vi "mirrors_and_piezo_manual_scan.vi"(1 "Stop Button":bool) -> ()   [LabVIEW 2013]
uses:
  <vilib>/Utility/error.llb/DialogType.ctl
  Piezo_micrometres_slider_control.ctl
  <vilib>/DAQmx/create/channels.llb/DAQmx Create Channel (AO-Voltage-Basic).vi
  <vilib>/DAQmx/create/channels.llb/DAQmx Create Channel (DO-Digital Output).vi
  <vilib>/DAQmx/write.llb/DAQmx Write (Analog DBL 1Chan 1Samp).vi
  <vilib>/DAQmx/write.llb/DAQmx Write (Digital Bool 1Line 1Point).vi
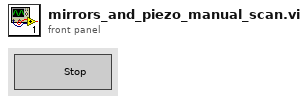
[diagram p1: front panel]
types:
  T1 = typedef "DialogType.ctl" = u16
  T2 = typedef "Piezo_micrometres_slider_control.ctl" = dbl
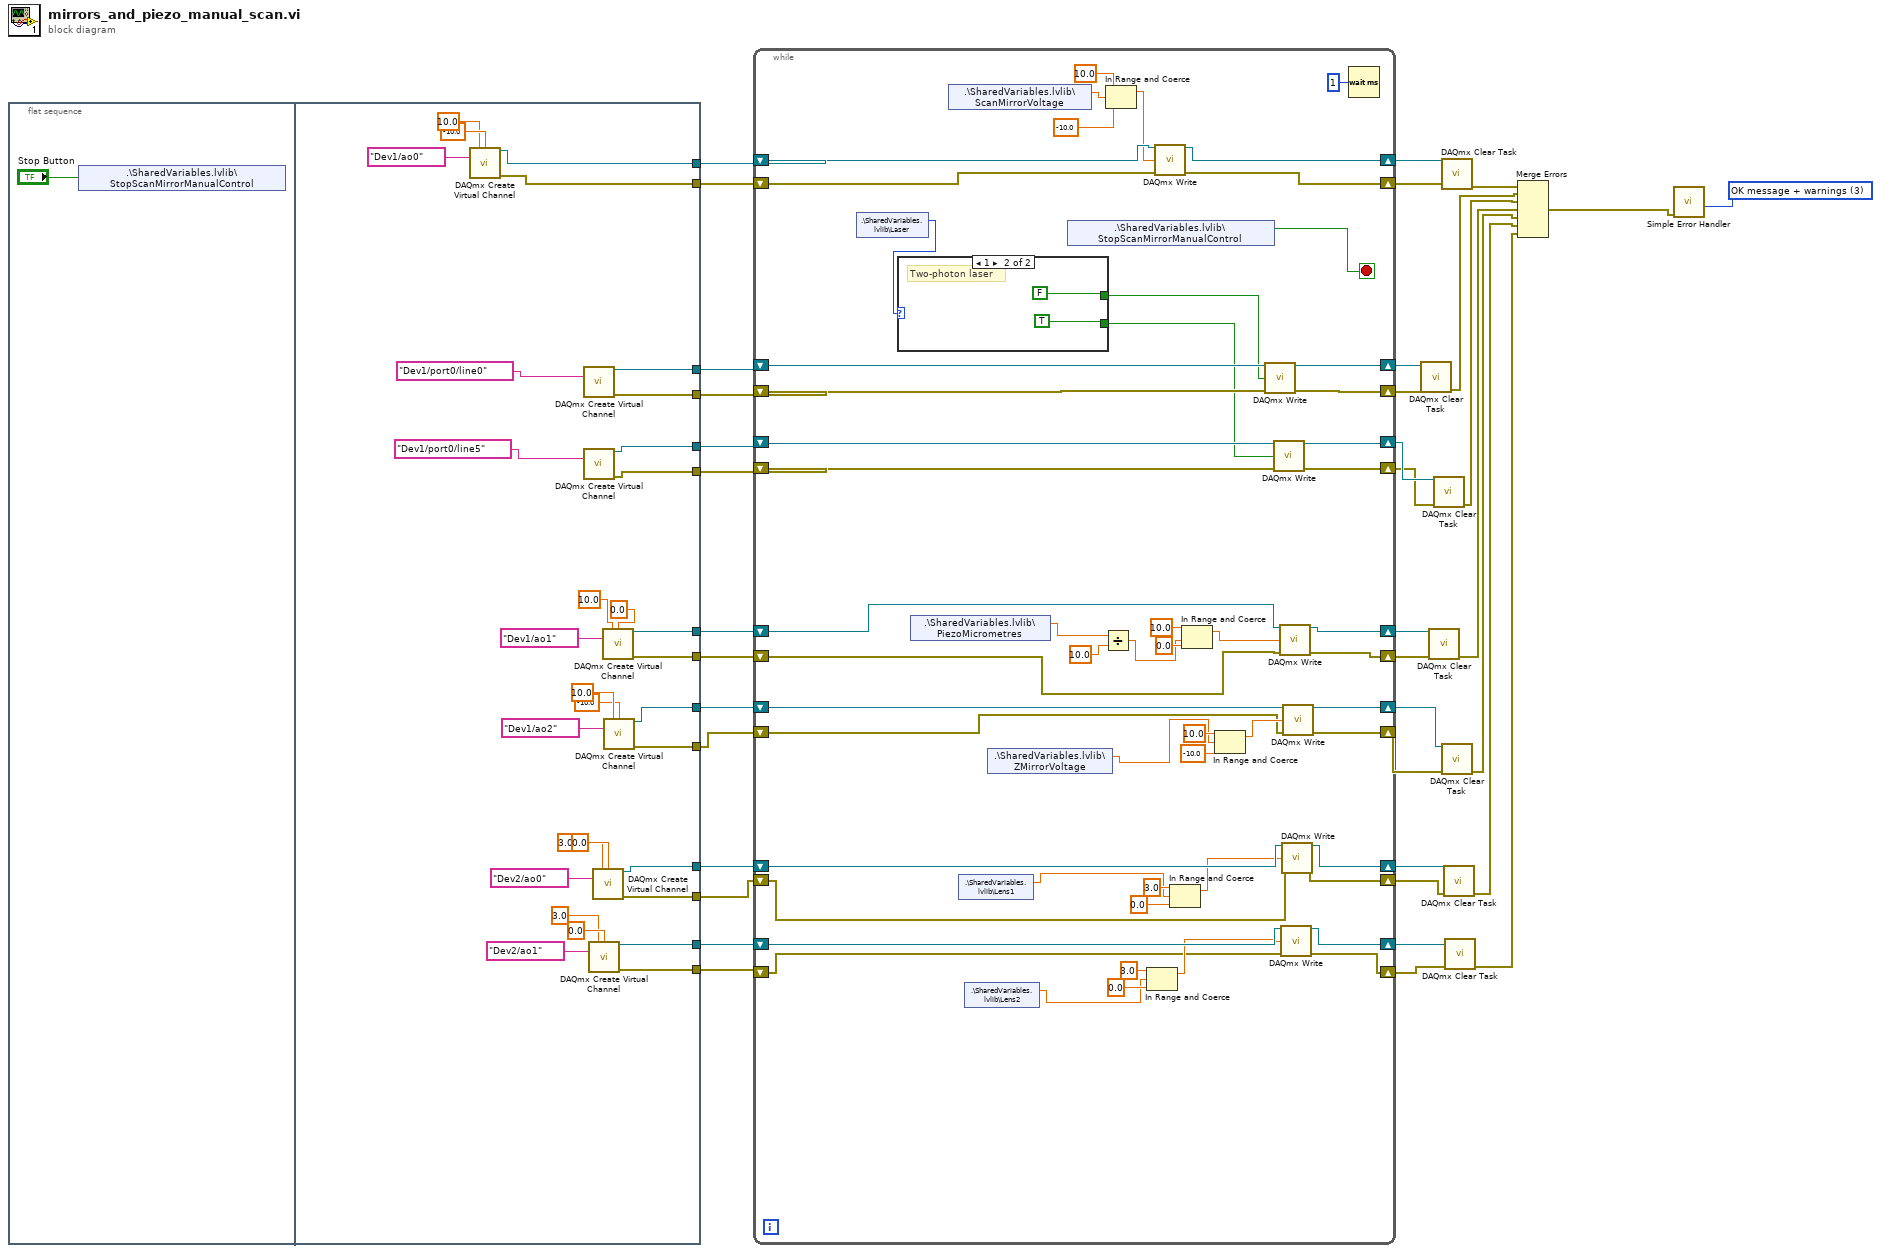
[diagram p0: block diagram]
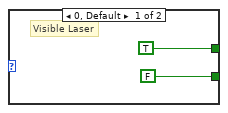
[diagram p2: hidden frame]
diagram:
  w21 = T1 3 items=["no dialog", "OK message", "continue or stop message", "OK message + warnings", "continue/stop + warnings"] ("type of dialog (OK msg:1)")
  n1 = flat-sequence {
    tunnel: [w66] -> w37
    tunnel: [w65] -> w36
    tunnel: [w64] -> w33
    tunnel: [w63] -> w32
    tunnel: [w62] -> w31
    tunnel: [w61] -> w30
    tunnel: [w52] -> w25
    tunnel: [w51] -> w24
    tunnel: [w50] -> w23
    tunnel: [w49] -> w22
    tunnel: [w48] -> w10
    tunnel: [w47] -> w5
    tunnel: [w46] -> w9
    tunnel: [w45] -> w4
    frame #0 {
      n2 = shared-variable ".\\SharedVariables.lvlib\\StopScanMirrorManualControl"("Stop Button") -> ()  [unwired: 1 in, 1 out]
    }
    frame #1 {
      n3 = call-poly <vilib>:"DAQmx Create Virtual Channel.vi"("maximum value"=10.0, "minimum value"=-10.0, "physical channels"=tag "Dev1/ao0") -> ("task out"=w66:refnum<k21>, "error out"=w65:errorcluster)  [unwired: 11 in]
      n4 = call-poly <vilib>:"DAQmx Create Virtual Channel.vi"("lines"=tag "Dev1/port0/line0" ("Physical Channel")) -> ("task out"=w64:refnum<k21>, "error out"=w63:errorcluster)  [unwired: 13 in]
      n5 = call-poly <vilib>:"DAQmx Create Virtual Channel.vi"("lines"=tag "Dev1/port0/line5") -> ("task out"=w62:refnum<k21>, "error out"=w61:errorcluster)  [unwired: 13 in]
      n6 = call-poly <vilib>:"DAQmx Create Virtual Channel.vi"("maximum value"=3.0, "minimum value"=0.0, "physical channels"=tag "Dev2/ao1") -> ("task out"=w46:refnum<k21>, "error out"=w45:errorcluster)  [unwired: 11 in]
      n7 = call-poly <vilib>:"DAQmx Create Virtual Channel.vi"("maximum value"=3.0, "minimum value"=0.0, "physical channels"=tag "Dev2/ao0") -> ("task out"=w48:refnum<k21>, "error out"=w47:errorcluster)  [unwired: 11 in]
      n8 = call-poly <vilib>:"DAQmx Create Virtual Channel.vi"("maximum value"=10.0, "minimum value"=0.0, "physical channels"=tag "Dev1/ao1") -> ("task out"=w52:refnum<k21>, "error out"=w51:errorcluster)  [unwired: 11 in]
      n9 = call-poly <vilib>:"DAQmx Create Virtual Channel.vi"("maximum value"=10.0, "minimum value"=-10.0, "physical channels"=tag "Dev1/ao2") -> ("task out"=w50:refnum<k21>, "error out"=w49:errorcluster)  [unwired: 11 in]
    }
  }
  n10 = while {
    shift-right: [w122] -> w34
    shift-left: w37 -> [w124]
    shift-right: [w121] -> w35
    shift-left: w36 -> [w123]
    shift-right: [w110] -> w29
    shift-left: w33 -> [w114]
    shift-right: [w109] -> w28
    shift-left: w32 -> [w113]
    shift-right: [w108] -> w27
    shift-left: w31 -> [w112]
    shift-right: [w107] -> w26
    shift-left: w30 -> [w111]
    shift-right: [w86] -> w17
    shift-left: w22 -> [w90]
    shift-right: [w87] -> w18
    shift-left: w23 -> [w91]
    shift-right: [w88] -> w19
    shift-left: w24 -> [w92]
    shift-right: [w89] -> w20
    shift-left: w25 -> [w93]
    shift-right: [w83] -> w8
    shift-left: w10 -> [w85]
    shift-right: [w82] -> w7
    shift-left: w9 -> [w84]
    shift-right: [w73] -> w6
    shift-left: w5 -> [w72]
    shift-right: [w70] -> w3
    shift-left: w4 -> [w71]
    stop <- w120 stop-if-true
    n11 = shared-variable ".\\SharedVariables.lvlib\\Laser"() -> (w104:u8)  [unwired: 1 in, 1 out]
    n12 = case shown="1" w104 {
      tunnel: [TRUE ("data") FALSE ("data")] -> w106
      tunnel: [FALSE ("data") TRUE ("data")] -> w105
      frame 0, Default {
        # "Visible Laser"
      }
      frame 1 {
        # "Two-photon laser"
      }
    }
    n13 = shared-variable ".\\SharedVariables.lvlib\\PiezoMicrometres"() -> (w95:dbl)  [unwired: 1 in, 1 out]
    n14 = shared-variable ".\\SharedVariables.lvlib\\ScanMirrorVoltage"() -> (w119:dbl)  [unwired: 1 in, 1 out]
    n15 = shared-variable ".\\SharedVariables.lvlib\\Lens1"() -> (w77:dbl)  [unwired: 1 in, 1 out]
    n16 = shared-variable ".\\SharedVariables.lvlib\\Lens2"() -> (w74:dbl)  [unwired: 1 in, 1 out]
    n17 = shared-variable ".\\SharedVariables.lvlib\\ZMirrorVoltage"() -> (w96:dbl)  [unwired: 1 in, 1 out]
    n18 = shared-variable ".\\SharedVariables.lvlib\\StopScanMirrorManualControl"() -> (w120:bool)  [unwired: 1 in, 1 out]
    n19 = Divide(x=w95, y=T2 10.0) -> (x/y=w94:T2)
    n20 = In Range and Coerce(upper limit=10.0, x=w119, lower limit=-10.0) -> (coerced(x)=w116:dbl)  [unwired: 1 out]
    n21 = In Range and Coerce(upper limit=3.0, x=w74, lower limit=0.0) -> (coerced(x)=w75:dbl)  [unwired: 1 out]
    n22 = call-poly <vilib>:"DAQmx Write.vi"("task/channels in"=w124, "data"=w116, "error in"=w123) -> ("task out"=w122:refnum<k21>, "error out"=w121:errorcluster)  [unwired: 10 in, 1 out]
    n23 = In Range and Coerce(upper limit=3.0, x=w77, lower limit=0.0) -> (coerced(x)=w76:dbl)  [unwired: 1 out]
    n24 = In Range and Coerce(upper limit=T2 10.0, x=w94, lower limit=T2 0.0) -> (coerced(x)=w97:T2)  [unwired: 1 out]
    n25 = In Range and Coerce(upper limit=10.0, x=w96, lower limit=-10.0) -> (coerced(x)=w98:dbl)  [unwired: 1 out]
    n26 = call-poly <vilib>:"DAQmx Write.vi"("task/channels in"=w114, "data"=w106, "error in"=w113) -> ("task out"=w110:refnum<k21>, "error out"=w109:errorcluster)  [unwired: 10 in, 1 out]
    n27 = call-poly <vilib>:"DAQmx Write.vi"("task/channels in"=w112, "data"=w105, "error in"=w111) -> ("task out"=w108:refnum<k21>, "error out"=w107:errorcluster)  [unwired: 10 in, 1 out]
    n28 = call-poly <vilib>:"DAQmx Write.vi"("task/channels in"=w93, "data"=w97, "error in"=w92) -> ("task out"=w89:refnum<k21>, "error out"=w88:errorcluster)  [unwired: 10 in, 1 out]
    n29 = call-poly <vilib>:"DAQmx Write.vi"("task/channels in"=w84, "data"=w75, "error in"=w71) -> ("task out"=w82:refnum<k21>, "error out"=w70:errorcluster)  [unwired: 10 in, 1 out]
    n30 = call-poly <vilib>:"DAQmx Write.vi"("task/channels in"=w85, "data"=w76, "error in"=w72) -> ("task out"=w83:refnum<k21>, "error out"=w73:errorcluster)  [unwired: 10 in, 1 out]
    n31 = call-poly <vilib>:"DAQmx Write.vi"("task/channels in"=w91, "data"=w98, "error in"=w90) -> ("task out"=w87:refnum<k21>, "error out"=w86:errorcluster)  [unwired: 10 in, 1 out]
    n32 = Wait (ms)(milliseconds to wait=u32 1) -> ()  [unwired: 1 out]
  }
  n33 = call <vilib>:"DAQmx Clear Task.vi"("task in"=w29, "error in"=w28) -> ("error out"=w14:errorcluster)  [unwired: 13 in]
  n34 = call <vilib>:"DAQmx Clear Task.vi"("task in"=w20, "error in"=w19) -> ("error out"=w12:errorcluster)  [unwired: 13 in]
  n35 = call <vilib>:"DAQmx Clear Task.vi"("task in"=w27, "error in"=w26) -> ("error out"=w13:errorcluster)  [unwired: 13 in]
  n36 = call <vilib>:"DAQmx Clear Task.vi"("task in"=w34, "error in"=w35) -> ("error out"=w15:errorcluster)  [unwired: 13 in]
  n37 = call <vilib>:"DAQmx Clear Task.vi"("task in"=w18, "error in"=w17) -> ("error out"=w11:errorcluster)  [unwired: 13 in]
  n38 = call <vilib>:"DAQmx Clear Task.vi"("task in"=w8, "error in"=w6) -> ("error out"=w2:errorcluster)  [unwired: 13 in]
  n39 = call <vilib>:"DAQmx Clear Task.vi"("task in"=w7, "error in"=w3) -> ("error out"=w1:errorcluster)  [unwired: 13 in]
  n40 = Merge Errors(w15, w14, w13, w12, w11, w2, w1) -> (w16:errorcluster)
  n41 = call <vilib>:"Simple Error Handler.vi"("type of dialog (OK msg:1)"=w21, "error in (no error)"=w16) -> ()  [unwired: 3 in, 5 out]
